vi "2023_day21_Task2.vi"() -> ()   [LabVIEW 2021]
uses:
  a007553b-196c-4698-b023-200d8bc566d7.vi
  <userlib>/_OpenG.lib/array/array.llb/Index 2D Array Elements (String)__ogtk.vi
  <userlib>/_OpenG.lib/array/array.llb/Search 1D Array (Boolean)__ogtk.vi
  <userlib>/_OpenG.lib/array/array.llb/Delete Elements from 2D Array (I32)__ogtk.vi
panel:
  out "Task 1":i32
  in  "Switch":bool caption="Ex. Data  vs.  User Data"
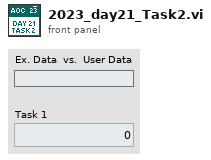
[diagram p1: front panel]
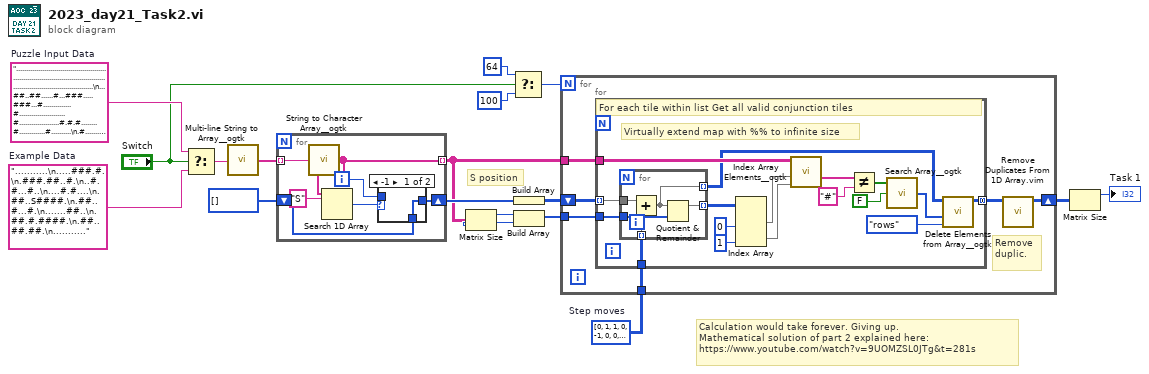
[diagram p0: block diagram]
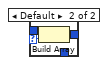
[diagram p2: hidden frame]
diagram:
  w11 = i32[][] [[0, 1], [1, 0], [-1, 0], [0, -1]]  # Step moves
  w17 = "...................................................................................................................................\n...##..##......#...###.....###...#..............#.......................#....................#.#.#........#.............#..........\n.#..........#...#.#..#....#.#........#.....#..#...........#..................................#.....#.............#..#.#.#.....##...\n..#....#...................#..........#....#..........#.#..........................#.............#.#.#..............#.#............\n....#...#............#....#.#.#..#.........#..#......#..#....................#..#.#.............##............#.............##.....\n..........#............##..#....#.#.............................#.................#....##.##.##....#...##..#.....#.....#.....#.....\n......#..#...#.#..............#.#......#.#.......#....#........##..#.......#.#.#.....#......#..#.#..#.......#.........##...........\n...#..#..............#....#.#.......#......#....#.....#.............#........................#.......#..#........#..........##.....\n...#....#...#..#..#.....#..#....#.#...#.....#...................#.............#...#.....#..#..#..#.........#.....#.......#.........\n....#....#.......##..........#............#..#.......................................#.#......#.#...#.....#...#........#...#.......\n.....#...###....#....#...#..............#.........................#.##......................##..#..#.#.##.........#...#............\n...........#.......#.......#.....#...............#................#.#..##...........##..#.......###.#.#..#...#.#..........#........\n..#......###..........#.#.......#..#..#..##....#...................#....#........###..#.#.....#...........#..............#..#....#.\n....#.........#.#....#.........#..#.#.....#...#.........#..#........#...................#....#.#....#..#.#.....#....#...##..#.##...\n....#..#....#.............#.......#.#...#..............#..........#....#...#........##...#.......#.........#.##............##......\n.......#.#...........#....#...................................#....#........#...........#.#.###...#.........#.##.#....#...#.#..##..\n....#..#........#..#..#.#..#.........#......#.............#..............#..................#.....#.#.....#..#.........#...#.......\n........##...##..#......##...........#.................#.....###..#....#...#..........#.#..............#..#......................#.\n.#............#.......##...........#.....................#.........#.........................##.....#..###.....#...#..###........#.\n...........##...#............#......#.................#.....#..#...#...#.......#.........#..##.........#....###.....#.#......##..#.\n.#....##.......#.......#...#..##..#.#...#............#.#...#......#...........................#.........#........#.........##......\n..#...#...##.#.......................##...........#..#........#.#.....##..#.##.#..#.......#..#.....#.####.#.......#......#.........\n.....#.##.#...##.#...........#.................#.....#....#.#..#.......#.........................#.#......#.##..#....#.#........#..\n.....##.###..#...................#.........................#..#....#..#....................................#..##..#.#...#..#..#.#..\n.#......#.#......#.............#.##..#.........##...##..........#.........#..#...#.#...........#.....##.......#.............##.#...\n....#..........#.#....#...#.#....................#.###.........#......##...#.........#............#........#....#..#....##.#...##..\n.............##.....#...#...#......#.............#............##.....#.......#.#........................#..#..........#...#........\n..#......##............#...#.........................##..##..............#..#......#.................##........#...............##..\n..#.......#...#......#...................#........#..#...##............##..#.....#..........................#.#..........#.........\n...##..#...##..........##....###.........#.......##..................#.......#....................#...........#.#........#.........\n......#....#......#.......#...#....................#..#........#..#......#..#.#....##.........................#.#....#.#....#....#.\n.....#......................#................#......##......##.#.........#..##.........#...............##.......#.........#........\n.#.#......#.#....#..#...#..............#......#..#.#.....#..........##.....#..#........#...#.#.........#..#.....................#..\n...#.##.#..#..#...#.#................###....................##.....#.#....#.........#......#..#..........##.#....#......#..#.......\n...#.................#.............#................#.................###..............#.................#..#......#.....#......##.\n.#.#.....#..#..........#...........#.#............#.##..#......#..##....#.#..###.......##.#.....#.........##...#.#...........#.....\n..#...#................#....................#..#..........#...............#.....#..#..####................#...............#........\n..........#..........#..............#........#...##...............#.....#...#...#..##.....#...#...........##.#.....##.#......#.....\n....#......#.......#...#.......#........#....#.....#..............#....#..##..#......#........#...............#.................#..\n.#.............#...............#...............#..#...#..#.#...#..#.......#....................#....#........#..##........#........\n.....................................#....###....#...#.....##.#.......#.........#.#.....#........#...........#...........##......#.\n.......#.##...#..............#..##..#...#...........#.##..##..#....#..#.........#........#.#.....................#.......#.......#.\n..#......##...................#..........#........##.....#..........#...#.#....#.#....#............##..............#...#.#.#.......\n...#.#.##.#.#.......................##......#.......#.........#.........#..........#........#.#.....#.#.............#.........#....\n.#.#...........#..................#....#......#.#............#....#.#..#...#..#..##.#............................#.#........#.##...\n..#...#....#...................#....#..........#.......................#.....##..#...#.#.#.......#...#..#.........#......##........\n.......#.................#...#........#....#.................#......................#...#.........##..................#......#.....\n..#..#....#..#...............#................#..#.#.....#.#..#.........###.......................#.#..#....#..........#...........\n......#...#..#...........#......................#..#............................#.....#........#.....##...#............#...........\n...........................##..#....#....#.....#....#....#...#........#.......#.........#.#..........##...#..................#..#..\n......#.....................#.....#.......#.#.....#.............#....#...#......#....#..#..........#........#...........#..........\n..#...#.............#..............#.#....#....#.....#....#...#.#......#.....#.#...........#.#.........#.#..................#..###.\n..#..............#....##......#.##..................#...##.........#..........#.................#..........#...................#...\n................#.##...#......##.........#.#...#..####.#.............#...#....#.........#.................................#........\n....#..........................#.......#...............#......#.......#...###.##.....#.#.#....#..###....#...#...##...........##....\n...#.#...............#..................#.........#...#.#..............#.....#.......#...#.##...#..#.......#.....#...........#.....\n.....#.....................#.#.#.....#.#.....#..#..##...#.....#...........#...##........#..#.......#.#...#....#..#............#....\n..#..........#....##..#.....###.#...............................#.#.##.#...#....##........#...#.....#....#............#.......#....\n.#...........#...#..#.....#..........#............#.......##......#.................#.#...#..##........#...............#...........\n.#................#........##.#.#.....#.#.............#.....#..#..##...............#..#................#.......#...#...##.......##.\n.#........#.##........##..#.#.##.....#..###..#......##...#......#..........#...............#.....#....#......#.....................\n............#.........#..............#.....#..#......................#...#.##.##...###..#..........###........###..................\n...........#...##.............#......#.....#.#...#...#.#..#....#..#............#....#..#.....#.#.........#.....#..#.###....#.......\n.........#........#.......#..#..##..#........#.#.#...........#....................##..#....#..#.....##.......##...##...............\n.......#....##..........##.....#...##....#.........#..#...................#......###.....#........#.....................#.#.#......\n.................................................................S.................................................................\n.....#...........#...#....#...#..#.........#.......##.#.............................#...#....#......#......#...#.#......#....#.....\n........###...#.......................#...........#.....#.#.........#.#......#...#.....#..#...###.....#.#....#..........#..........\n...............#.#............#.#......#...#..#.......#..#.#..#....##.#..#....#...............#.##.#..#...#...#..#.................\n.............#.##..........#........#.#........###.....#..............#.......#..........##...........#........#...#...............\n...........#.#.#........#......###.....#.#......#.#..##..#..#...#...##.#.#...##.......#........#..#.#.##...###...........#.........\n..........##..............#......#.............#..#.#....#..#.....#.#...#..........##............#...#.##.....#.#..#...............\n.#.#...............#.#............##.......#...#..#....#.....#........#.#..###...#.....#.........#................#..#.............\n.............#...#........#....#....#..........##.#....#......#.....#.........#..#........#.......###....#.#....#....##............\n...#............#.#......#...#....#..............#.....#..##....#.....#....#.....#...#...#.#..#.........#.#.........#..............\n..............#.......#...........#..............#.#.......#..#.#......#...##.......#................#...#.....#...#...............\n...##...........................#...#...#.......#............#.#.....#...#....#..#......#..#.##....#.#...#...#.................#.#.\n...#....#...........#.........##...#............#...............#...................................##..#......#..#..............#.\n...##.#.#.............#....#.##.#........#.....#.#...#.....##...........#.....................#...#..#......#............##.....#..\n...#..#...#...............#.#......#....#.#.#......#...................#......#.....##....#....#....##...#......#..............#...\n......#..#.........#.................#...#................#.........#..................................................#....#......\n.#..........#..........#..................#.#...#....#....#.#.........#..#...#........#......#.............#....................#..\n........#............#........#.......##......##....#................#.......#....#.#.....#............#.#.#...............###.....\n.##........#..........#...#......##..#.##.#.....##.........................#.....##.#...#......#.#......#..#..........#............\n....#....................#...#.......#...#.......#.....#......#...#..#...#......#.#..#...##.##..#.....##...........#..#.###........\n.#.....#........#..............#...#...#.........#.#................#.#.............##.#....#..#.....................#.....#..###..\n......#...#.#..#.............##.#........#.....................#........#....#...........#....##......................#............\n..#.....##...#..#.#.........#.#.......#.#..#......#..........#.##....#..#..................#.........#..#........#....##...........\n..#...#.#....#.#...................##......##...........#...#.............#..........#.##..#.#......#..................#..#.#...##.\n...##...#........#.#.........#...#.....#.#...##...#...#..#.#.........#.....#..#....#.###...#........#.............#.........#....#.\n.........#...#.#...#.#.................#............#........................#.#.....#.........#................#.....#..#......#..\n...........#.#..#.............##........#..........#....#...........#....#.....#....#....#.#......##.........#..##....#..##........\n.........#..................................#..#...............#...#..#...#...#..#......#.#..#.............#...........#.#..#...##.\n.#.#......#..#.......#.##........#......#....#................#...#...##..##....#.....#..........#.........#....#..#.#.........#...\n.....#.....#.........#............#....#.....................#....#.##...#......................#................#.#.#...#.........\n.....#.............##..#..........#..#..............##..#.................##........###.....#.#.........#.#.#...............#......\n.#.#.#...#.#..............#...............#...............#..#.....#......#..............................#.......#.#...#.#...#.....\n.................#........#...............#.........................................#......................#....#............#...#.\n.#...#.###...........#...#..##...............#.........#...##....................#...........#...............#....##...........#.#.\n..###...#.#.........##.................#.#.....#..##...........#....##........#...#...................##..##...#................#..\n...#.................#.....#...........#....#...##...#.......#............#.....#.#........#........#...#...##...#.##..............\n.......#....#.........#.#.....#.#.......#.....#....#...#.............#.....#.....#.##.....................#.###...........#........\n................#....#..#.......#.............#......#.......#.................#.#................#..........#.....##...#..#....#..\n........#...#...#.#......##......#.........#.......................#.........#...#.....................#..........#.#..#...#.......\n....#.......##......##....##.................#.....#.#.#....#...#...........#.......................#........#....#....#.....#...#.\n.#..##..##.........#......#.........#.......#....#....#...#.....#..#.....#.#............................#...#..................#.#.\n...#......#............##.....##.............##.................#..#....#.#...#....#......................##....#.....#........#...\n........#....#....#..........#.###....#................#..##......#..#...#..#......#..........##...............#..#.........#...#..\n.....#...#.##.....#....#.##.........#............##....#..#.#.....#.............#...................#..#............#..#..#.#....#.\n.....#..#.........##..#...........#....#............#.#...........#..............##.......#.#...........#..####.....##.#.##........\n...#.#.#.##.#.#..#.....#........###..#............#........##......##.#..........................####........##.#.....#......#.....\n.##.#.#...##..#........##....#........#............#...#...#......#....#....##..#...........#.#.........#.##...#...#...#...#.#.....\n......#.#..#.#........##.#....#.#...#.###..#...........#...................#.................#.#.#............##.#...#.#.........#.\n........#.#....#...#...#..........#.#..#..#...........#..#...#.....##......#.....................##..#........#.....#.#.....#....#.\n..#.......##....##............##...............................#......#.#..#.............#..........................#....#.........\n.......#....#................#...........#...##................#...#.#....#...............#....##.......................#.#.....#..\n..........#...........#..#..#.....#...........##...........#......#.#.#.#..........#..........#.....#......................###.....\n....#.......##...........#..........#..###.#.........................#....#..........#.#.........#......#............#..#.....#..#.\n...#.#...#...#.............#.......#...#.##..............................#........##.......##..#...#......................#........\n...........##.............#....##....#.#...#.#..............#..#..................#.......#......#.......#.................#..#....\n.#.##..#......#...#..#........#.......#.#.#....#...............#........................#..........#...............................\n........#...........#....#...#...##..#.#....###................#...#.................#..................#.......#....#........#..#.\n.........#.###.#....#..#..##..........#.#.......#............................#..##....#.....#....#....#.#...##......##.............\n..#.#..##.#........#..#.#...#........#...#...#.....................##...........#.....#...#.#.#...#.......#..#..#.........#..#..#..\n.....#..........####....##..##......#.............#...#...........#........#..........#.............###...#.#.#...#................\n..#.....#...#....#.#.........#....#..#.......##.....#.............#........#............#...###.........#...#......................\n.##..............#..#....#..#......#....##..#......#.###.#..................#...............#.#..#..#.##..........#............#.#.\n..#..#..#.....................#.#..............##...#.....#....................#..##...#.........#...........#..##.........#....#..\n....#...............#.......#.#....##....#..#..........................#.......#.##...........#.......#....#.#........#..#.........\n.....##.......#.................................#........#..................#..#.#......#....#..#....#...#.........................\n..................................................................................................................................."  # Puzzle Input Data
  w18 = "...........\n.....###.#.\n.###.##..#.\n..#.#...#..\n....#.#....\n.##..S####.\n.##..#...#.\n.......##..\n.##.#.####.\n.##..##.##.\n..........."  # Example Data
  # "Calculation would take forever. Giving up.\nMathematical solution of part 2 explained here:\nhttps://www.youtube.com/watch?v=9UOMZSL0JTg&t=281s"
  # "S position"
  n1 = Select(t=w17, s="Switch", f=w18) -> (s? t:f=w16:string)
  n2 = call <userlib>:"Multi-line String to Array__ogtk.vi"("string"=w16) -> ("lines"=w15:string[])
  n3 = for {
    tunnel: w15 -> [w25] mode=indexing
    tunnel: [w24] -> w2 mode=indexing
    shift-right: [w20] -> w13
    shift-left: i32[] [] -> [w19]
    i -> [w21]
    n4 = call <userlib>:"String to Character Array__ogtk.vi"("Input String"=w25) -> ("Character Array"=w24:string[])
    n5 = Search 1D Array(1D array=w24, element="S") -> (index of element=w22:i32)  [unwired: 1 in]
    n6 = case shown="-1" w22 {
      selector: w22 -> [_ w29]
      tunnel: w21 -> [_ w28]
      tunnel: [w26 w27] -> w20
      tunnel: w19 -> [w26 _]
      frame -1 {
      }
      frame Default {
        n7 = Build Array(w28, w29) -> (w27:i32[])
      }
    }
  }
  n8 = Matrix Size(0:w2) -> (1:w4:i32, 2:w3:i32)
  n9 = Select(t=64, s="Switch", f=100) -> (s? t:f=w6:i32)
  n10 = Build Array(w13) -> (w12:i32[][])
  n11 = Build Array(w4, w3) -> (w1:i32[])
  n12 = for {
    N: w6 -> [_]
    tunnel: w2 -> [w34]
    shift-right: [w31] -> w10
    shift-left: w12 -> [w33]
    tunnel: w11 -> [w35]
    tunnel: w1 -> [w30]
    # "Remove duplic."
    n13 = for {
      tunnel: w33 -> [w51] mode=indexing
      tunnel: w35 -> [w52]
      tunnel: w34 -> [w50]
      tunnel: [w39] -> w32 mode=concatenating
      tunnel: w30 -> [w37]
      # "Virtually extend map with %% to infinite size"
      # "For each tile within list Get all valid conjunction tiles"
      n14 = for {
        tunnel: w52 -> [w57] mode=indexing
        tunnel: w51 -> [w56]
        tunnel: [w54] -> w42 mode=indexing
        tunnel: w37 -> [w55]
        tunnel: [w53] -> w36 mode=indexing
        n15 = Add(x=w56, y=w57) -> (x+y=w53:i32[])
        n16 = Quotient & Remainder(x=w53, y=w55) -> (x-y*floor(x/y)=w54:i32[])  [unwired: 1 out]
      }
      n17 = Index Array(array=w42, index (col) #1=0 ("index (row)"), index (col) #2=1 ("index (row)")) -> (element #1=w47:i32[], element #2=w46:i32[])  [unwired: 2 in]
      n18 = call-poly <userlib>:"Index Array Elements__ogtk.vi"("indices 1"=w46, "indices 0"=w47, "array"=w50) -> ("elements"=w48:string[])  [unwired: 8 in]
      n19 = Not Equal?(x=w48, y="#" ("element")) -> (x != y?=w38:bool[])
      n20 = call-poly <userlib>:"Search Array__ogtk.vi"("Array"=w38, "Element Data"=FALSE) -> ("Indices of Elements"=w41:i32[])  [unwired: 7 in]
      n21 = call-poly <userlib>:"Delete Elements from Array__ogtk.vi"("delete (rows or columns)"=enum16{"rows", "columns"}."rows", "indices"=w41, "array"=w36) -> ("array w/ subset deleted"=w39:i32[][])  [unwired: 7 in, 1 out]
    }
    n22 = call "Remove Duplicates From 1D Array.vim"("array"=w32) -> ("array with duplicates removed"=w31:i32[][])  [unwired: 10 in]
  }
  n23 = Matrix Size(0:w10) -> (1:→"Task 1":i32)  [unwired: 1 out]
